vi "Practica5.2_Event.vi"() -> ()   [LabVIEW 2022 SP3]
panel:
  out "Aún NO":bool
  out "Prueba":bool
  out "Activado":bool
  in  "Selector":bool
  # "Anahí Montserrat Vázquez Padilla \nPráctica 05: Event\n13/02/2024"
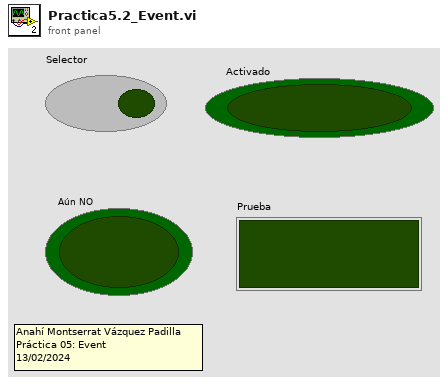
[diagram p1: front panel]
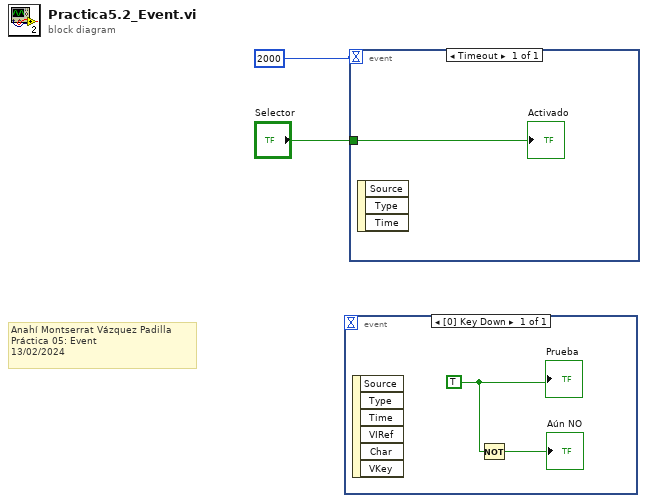
[diagram p0: block diagram]
diagram:
  # "Anahí Montserrat Vázquez Padilla \nPráctica 05: Event\n13/02/2024"
  n1 = event shown="[0] Key Down" {
    selector: _ -> [_]
    dyn-events: _ -> [_]
    timeout: _ -> [_]
    event Key Down {
      w3 = TRUE
      n2 = event-data() -> ()  [unwired: 1 in, 6 out]
      n3 = Not(x=w3) -> (.not. x?=→"Aún NO":bool)
      "Prueba" <- w3
    }
  }
  n4 = event shown="[0] Timeout" {
    selector: _ -> [_]
    dyn-events: _ -> [_]
    timeout: 2000 -> [_]
    tunnel: "Selector" -> [w5]
    event Timeout {
      n5 = event-data() -> ()  [unwired: 1 in, 3 out]
      "Activado" <- w5
    }
  }
